vi "Auto_Drive.vi"(8 "Timer?":bool, 9 "Duration":u32=3500, 10 "distance":dbl=88.0 format="%#_13g", 11 "Drive Effort":dbl=1000.0) -> ()   [LabVIEW 2016]
uses:
  <vilib>/Rock Robotics/WPI/SafetyOutput/WPI_SafetyOutputConfigMenu.ctl
panel:
  out "Encoder Difference":dbl
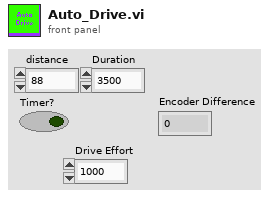
[diagram p1: front panel]
types:
  T1 = typedef "WPI_SafetyOutputConfigMenu.ctl" = enum16{"Enable", "Disable"}
  T2 = typedef "WPI_MotorControlDeviceRef.ctl" = cluster{"DeviceStatus":errorcluster, "Type":T3, "PWM":cluster{"PWM Channel":T4, "DeadBand":T5}, "CAN":cluster{"Device Number":u8, "SetOutput VI Ref":variant, "GetOutput VI Ref":variant, "Enable VI Ref":variant, "Disable VI Ref":variant, "Data":variant}, "Invert":bool}
  T3 = typedef "WPI_MotorControlType.ctl" = enum16{"PWM", "CAN"}
  T4 = typedef "FPGA_DIOPWMChannel.ctl" = enum8{"PWM 0", "PWM 1", "PWM 2", "PWM 3", "PWM 4", "PWM 5", "PWM 6", "PWM 7", "PWM 8", "PWM 9", "PWM MXP 0", "PWM MXP 1", "PWM MXP 2", "PWM MXP 3", "PWM MXP 4", "PWM MXP 5", "PWM MXP 6", "PWM MXP 7", "PWM MXP 8", "PWM MXP 9", "Invalid"}
  T5 = typedef "WPI_PWMDeadband.ctl" = cluster{"Name":string, "maxPositivePwm":i32, "minPositivePwm":i32, "centerPwm":i32, "maxNegativePwm":i32, "minNegativePwm":i32, "angularRange":u16}
  T6 = typedef "WPI_CANTalonSRX_GlobalStatus.ctl" = cluster{"Applied Throttle":dbl, "Module Enabled":bool, "CAN Error":errorcluster, "Closed Loop Error":dbl, "Forward Limit Switch Closed":bool, "Reverse Limit Switch Closed":bool, "Sensor Position":dbl, "Sensor Velocity":dbl, "Current":dbl, "Sticky Fault - Over Temp":bool, "Sticky Fault - Under Voltage":bool, "Sticky Fault - Forward Limit":bool, "Sticky Fault - Reverse Limit":bool, "Sticky Fault - Forward Soft Limit":bool, "Sticky Fault - Reverse Soft Limit":bool, "Brake is Enabled":bool, "Encoder Position":dbl, "Encoder Velocity":dbl, "Encoder Index Count":dbl, "Encoder A Pin State":bool, "Encoder B Pin State":bool, "Encoder Index Pin State":bool, "Analog In":dbl, "Analog In Velocity":dbl, "Temperature (C)":dbl, "Battery Voltage":dbl, "Control 5 Is Supported":bool, "Current Profile Slot Select":dbl, "Pos Div 8":bool, "Vel Div 4":bool, "Pulse Width Position":i32, "Pulse Width Velocity":i32, "Pulse Width Rise To Rise (us)":i32, "Pulse Width Rise To Fall (us)":i32, "Mot Prof Active Is Under Run":bool, "Mot Prof Active Has Under Run":bool, "Mot Prof Active Is Last":bool, "Mot Prof Active Velocity Only":bool, "Mot Prof Active Is Valid":bool, "Mot Prof Buffer Is Full":bool, "Mot Prof Active Profile Slot Select":i32, "Mot Prof NextID":i32, "Mot Prof Count":i32, "Mot Prof Active Velocity":dbl, "Mot Prof Active Position":dbl, "Mot Prof Output Enable":i32}
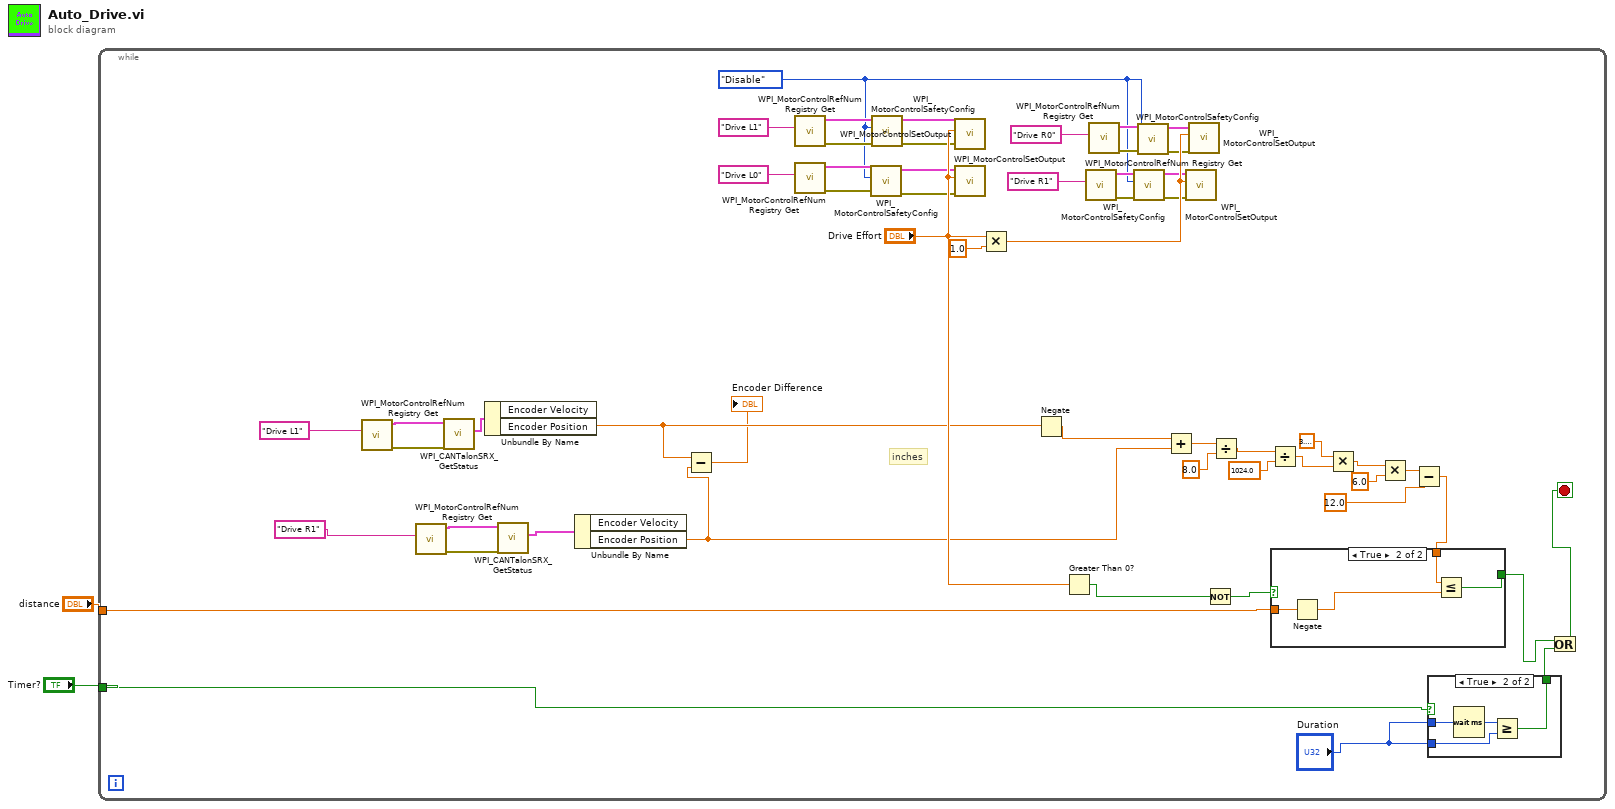
[diagram p0: block diagram]
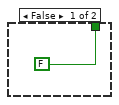
[diagram p2: hidden frame]
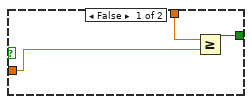
[diagram p3: hidden frame]
diagram:
  n1 = while {
    tunnel: "distance" -> [w38]
    tunnel: "Timer?" -> [w33]
    stop <- w27 stop-if-true
    w6 = WPI_SafetyOutputConfigMenu."Disable" ("mode")
    # "inches"
    n2 = call <vilib>:"WPI_MotorControlRefNum Registry Get.vi"("refnum name"="Drive L1") -> ("error out"=w50:errorcluster, "MotorControlDevRef"=w55:T2)  [unwired: 9 in]
    n3 = call <vilib>:"WPI_MotorControlRefNum Registry Get.vi"("refnum name"="Drive R1") -> ("error out"=w53:errorcluster, "MotorControlDevRef"=w54:T2)  [unwired: 9 in]
    n4 = call <vilib>:"WPI_CANTalonSRX_GetStatus.vi"("error in (no error)"=w50, "CAN Talon SRX Ref"=w55) -> ("Talon SRX Status"=w52:T6)  [unwired: 7 in, 2 out]
    n5 = Unbundle By Name(w52) -> ("Encoder Position"=w5:dbl)  [unwired: 1 out]
    n6 = call <vilib>:"WPI_CANTalonSRX_GetStatus.vi"("error in (no error)"=w53, "CAN Talon SRX Ref"=w54) -> ("Talon SRX Status"=w51:T6)  [unwired: 7 in, 2 out]
    n7 = Unbundle By Name(w51) -> ("Encoder Position"=w4:dbl)  [unwired: 1 out]
    n8 = Subtract(x=w5, y=w4) -> (x-y=→"Encoder Difference":dbl)
    n9 = call <vilib>:"WPI_MotorControlRefNum Registry Get.vi"("refnum name"="Drive L1") -> ("error out"=w21:errorcluster, "MotorControlDevRef"=w22:T2)  [unwired: 9 in]
    n10 = call <vilib>:"WPI_MotorControlRefNum Registry Get.vi"("refnum name"="Drive L0") -> ("error out"=w17:errorcluster, "MotorControlDevRef"=w18:T2)  [unwired: 9 in]
    n11 = call <vilib>:"WPI_MotorControlSafetyConfig.vi"("error in (no error)"=w17, "mode"=w6, "MotorControlDevRef"=w18) -> ("error out"=w15:errorcluster, "MotorControlDevRef"=w16:T2)  [unwired: 7 in]
    n12 = call <vilib>:"WPI_MotorControlSafetyConfig.vi"("error in (no error)"=w21, "mode"=w6, "MotorControlDevRef"=w22) -> ("error out"=w19:errorcluster, "MotorControlDevRef"=w20:T2)  [unwired: 7 in]
    n13 = call <vilib>:"WPI_MotorControlSetOutput.vi"("error in (no error)"=w19, "Output"="Drive Effort", "MotorControlDevRef"=w20) -> ()  [unwired: 6 in, 3 out]
    n14 = call <vilib>:"WPI_MotorControlSetOutput.vi"("error in (no error)"=w15, "Output"="Drive Effort", "MotorControlDevRef"=w16) -> ()  [unwired: 6 in, 3 out]
    n15 = Multiply(x="Drive Effort", y=1.0) -> (x*y=w24:dbl)
    n16 = Negate(x=w5) -> (-x=w49:dbl)
    n17 = Greater Than 0?(x="Drive Effort") -> (x > 0?=w34:bool)
    n18 = call <vilib>:"WPI_MotorControlRefNum Registry Get.vi"("refnum name"="Drive R1") -> ("error out"=w9:errorcluster, "MotorControlDevRef"=w10:T2)  [unwired: 9 in]
    n19 = call <vilib>:"WPI_MotorControlRefNum Registry Get.vi"("refnum name"="Drive R0") -> ("error out"=w13:errorcluster, "MotorControlDevRef"=w14:T2)  [unwired: 9 in]
    n20 = call <vilib>:"WPI_MotorControlSafetyConfig.vi"("error in (no error)"=w9, "mode"=w6, "MotorControlDevRef"=w10) -> ("error out"=w8:errorcluster, "MotorControlDevRef"=w7:T2)  [unwired: 7 in]
    n21 = call <vilib>:"WPI_MotorControlSafetyConfig.vi"("error in (no error)"=w13, "mode"=w6, "MotorControlDevRef"=w14) -> ("error out"=w12:errorcluster, "MotorControlDevRef"=w11:T2)  [unwired: 7 in]
    n22 = Add(x=w49, y=w4) -> (x+y=w48:dbl)
    n23 = call <vilib>:"WPI_MotorControlSetOutput.vi"("error in (no error)"=w8, "Output"=w24, "MotorControlDevRef"=w7) -> ()  [unwired: 6 in, 3 out]
    n24 = call <vilib>:"WPI_MotorControlSetOutput.vi"("error in (no error)"=w12, "Output"=w24, "MotorControlDevRef"=w11) -> ()  [unwired: 6 in, 3 out]
    n25 = Not(x=w34) -> (.not. x?=w25:bool)
    n26 = Divide(x=w48, y=8.0) -> (x/y=w46:dbl)
    n27 = Divide(x=w46, y=1024.0) -> (x/y=w44:dbl)
    n28 = Multiply(x=3.141592653589793, y=w44) -> (x*y=w42:dbl)
    n29 = Multiply(x=w42, y=6.0) -> (x*y=w37:dbl)
    n30 = Subtract(x=w37, y=12.0) -> (x-y=w35:dbl)
    n31 = case shown="True" w25 {
      tunnel: [w63 w69] -> w29
      tunnel: w38 -> [w64 w67]
      tunnel: w35 -> [w65 w66]
      frame False {
        n32 = Greater Or Equal?(x=w65, y=w64) -> (x >= y?=w63:bool)
      }
      frame True {
        n33 = Negate(x=w67) -> (-x=w68:dbl)
        n34 = Less Or Equal?(x=w66, y=w68) -> (x <= y?=w69:bool)
      }
    }
    n35 = case shown="True" w33 {
      tunnel: "Duration" -> [_ w61]
      tunnel: [FALSE w60] -> w28
      tunnel: "Duration" -> [_ w59]
      frame False {
      }
      frame True {
        n36 = Wait (ms)(milliseconds to wait=w59) -> (millisecond timer value=w62:u32)
        n37 = Greater Or Equal?(x=w62, y=w61) -> (x >= y?=w60:bool)
      }
    }
    n38 = Or(x=w29, y=w28) -> (x .or. y?=w27:bool)
  }
